vi "espectro_hz.vi"(9 "fs":dbl, 10 "N FFT":i32, 11 "X":dbl[](array[numeric])) -> (2 "XScale":dbl, 3 "FFT(X)":cdb[](array[numeric]))   [LabVIEW 2020]
uses:
  <vilib>/Analysis/2dsp.llb/Real FFT.vi
  <vilib>/Analysis/NI_AALPro.lvlib
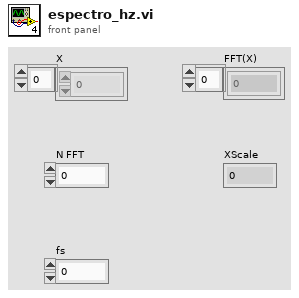
[diagram p1: front panel]
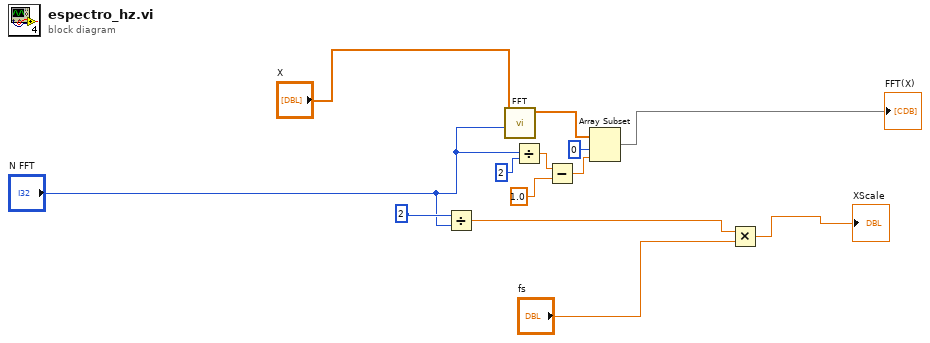
[diagram p0: block diagram]
diagram:
  n1 = Divide(x=2, y="N FFT") -> (x/y=w10:dbl)
  n2 = call-poly <vilib>:"FFT.vi"("FFT size"="N FFT", "X"="X") -> ("FFT {X}"=w4:cdb[])  [unwired: 8 in, 1 out]
  n3 = Divide(x="N FFT", y=2) -> (x/y=w3:dbl)
  n4 = Subtract(x=w3, y=1.0) -> (x-y=w1:dbl)
  n5 = Array Subset(array=w4, index=0, length=w1) -> (→"FFT(X)":cdb[])
  n6 = Multiply(x=w10, y="fs") -> (x*y=→"XScale":dbl)
